vi "motor_write_then_read.vi"(4 "Error in":errorcluster, 5 "Semaphore in":T1, 6 "Data to write":string, 7 "VISA resource name in":refnum<visa-resource-name>) -> (0 "Error out":errorcluster, 1 "Semaphore out":T1, 2 "Received data":string, 3 "VISA resource name out":refnum<visa-resource-name>)   [LabVIEW 2010]
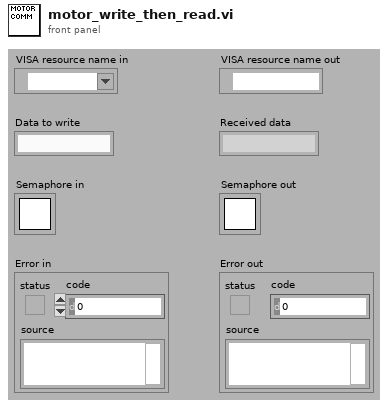
[diagram p1: front panel]
types:
  T1 = typedef "Semaphore RefNum" = refnum<k1>
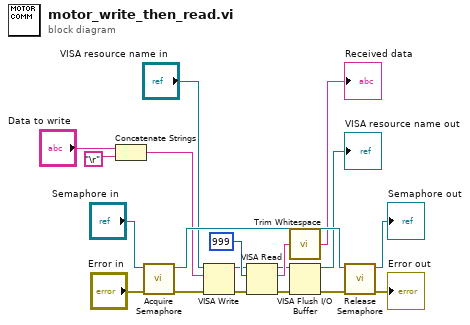
[diagram p0: block diagram]
diagram:
  n1 = Concatenate Strings("Data to write", "\r") -> (w7:string)
  n2 = call <vilib>:"Acquire Semaphore.vi"("error in (no error)"="Error in", "semaphore"="Semaphore in") -> ("error out"=w18:errorcluster, "semaphore out"=w15:T1)  [unwired: 3 in, 1 out]
  n3 = VISA Write(VISA resource name="VISA resource name in", write buffer=w7, error in (no error)=w18) -> (VISA resource name out=w3:refnum<visa-resource-name>, error out=w4:errorcluster)  [unwired: 1 out]
  n4 = VISA Read(VISA resource name=w3, byte count=u32 999, error in (no error)=w4) -> (VISA resource name out=w2:refnum<visa-resource-name>, read buffer=w11:string, error out=w1:errorcluster)  [unwired: 1 out]
  n5 = call <vilib>:"Trim Whitespace.vi"("string"=w11) -> ("trimmed string"=→"Received data":string)  [unwired: 1 in]
  n6 = VISA Flush I/O Buffer(VISA resource name=w2, error in (no error)=w1) -> (VISA resource name out=→"VISA resource name out":refnum<visa-resource-name>, error out=w13:errorcluster)  [unwired: 1 in]
  n7 = call <vilib>:"Release Semaphore.vi"("error in (no error)"=w13, "semaphore"=w15) -> ("error out"=→"Error out":errorcluster, "semaphore out"=→"Semaphore out":T1)  [unwired: 4 in]
